vi "VCS Get Interface Name.vi"(8 "error in (no error)":errorcluster, 11 "axis in":cluster{"keyHandle":u32, "nodeId":u16}={"keyHandle"=0, "nodeId"=1}) -> (0 "error out":errorcluster, 2 "interfaceName":string, 3 "axis out":cluster{"keyHandle":u32, "nodeId":u16}={"keyHandle"=0, "nodeId"=1})   [LabVIEW 2010]
doc: "<B>VCS Get Interface Name</B> returns the interface name to corresponding handle."
uses:
  Resources/EposCmd.dll
  Resources/EposCmd64.dll
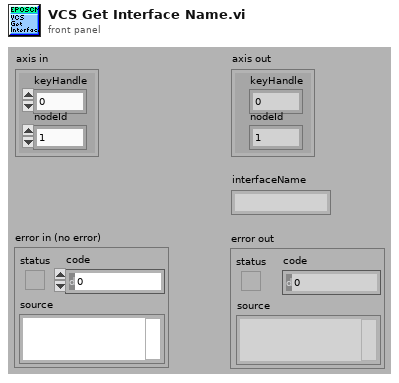
[diagram p1: front panel]
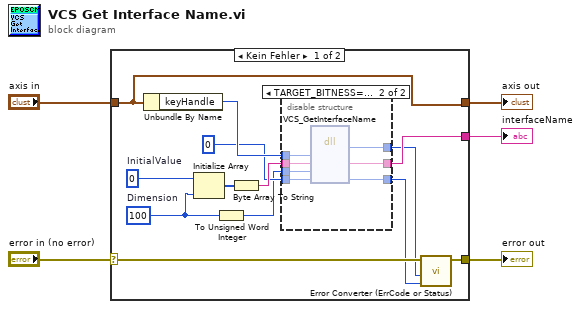
[diagram p0: block diagram]
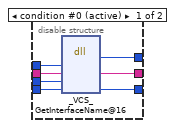
[diagram p2: hidden frame]
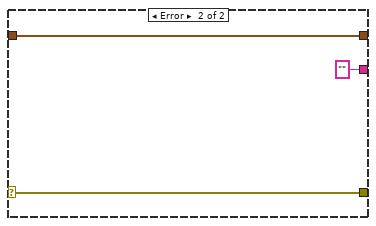
[diagram p3: hidden frame]
diagram:
  n1 = case shown="Kein Fehler" "error in (no error)" {
    selector: "error in (no error)" -> [w17 w35]
    tunnel: [w16 w35] -> w4
    tunnel: [w18 "" ("pInterfaceName")] -> w3
    tunnel: "axis in" -> [w9 w34]
    tunnel: [w9 w34] -> w1
    frame No Error {
      w12 = u8 0  # InitialValue
      w7 = 100  # Dimension
      n2 = Unbundle By Name(w9) -> ("keyHandle"=w14:u32)
      n3 = Initialize Array(w12, w7) -> (w13:u8[])
      n4 = To Unsigned Word Integer(number=w7) -> (unsigned 16bit integer=w6:u16)
      n5 = Byte Array To String(unsigned byte array=w13) -> (string=w11:string)
      n6 = disable-structure shown="TARGET_BITNESS==64" {
        disable-tunnel: [w25 w32] -> w18
        disable-tunnel: [w24 w31] -> w15
        disable-tunnel: w14 -> [w23 w30]
        disable-tunnel: w11 -> [w22 w29]
        disable-tunnel: w6 -> [w21 w28]
        disable-tunnel: u32 0 ("pErrorCode") -> [w20 w27]
        disable-tunnel: [w19 w26] -> w8
        frame condition #0 (active) {
          n7 = dll-call lib="C:/Sources/LabView/maxon EPOS/Resources/EposCmd.*" fn="_VCS_GetInterfaceName@16"("KeyHandle"=w23, "pInterfaceName"=w22, "MaxStrSize"=w21, "pErrorCode"=w20) -> (w19:i32, "pInterfaceName"=w25:string, "pErrorCode"=w24:u32)  [unwired: 5 in, 2 out]
        }
        frame condition #1 {
          n8 = dll-call lib="C:/setup/Resources/EposCmd64.dll" fn="VCS_GetInterfaceName" ("EposCmd.dll:_VCS_GetInterfaceName@16")("KeyHandle"=w30, "pInterfaceName"=w29, "MaxStrSize"=w28, "pErrorCode"=w27) -> ("Rückgabetyp"=w26:i32, "pInterfaceName"=w32:string, "pErrorCode"=w31:u32)  [unwired: 5 in, 2 out]
        }
      }
      n9 = call "Error Converter (ErrCode or Status).vi"("error code"=w15, "return type"=w8, "error in (no error)"=w17) -> ("error out"=w16:errorcluster)  [unwired: 7 in]
    }
    frame Error {
    }
  }
  "interfaceName" <- w3
  "error out" <- w4
  "axis out" <- w1
